vi "SP Convert Markers From Points.vi"(10 "Sweep":T8, 11 "Plot Control In":T1={"Trace Orientation"=enum."Overlay", "Frequency"={"Change Frequency"=FALSE, "Start"=500.0, "Stop"=1500.0, "Units"=enum."MHz"}, "Markers"=[], "Traces"=[]} {"Traces"."Reference" format="%#.2g"; "Traces"."Display Data" items=["Data", "Memory", "Data/Memory"]; "Traces"."Format" items=["Log Mag", "Phase", "Expanded Phase", "Delay", "Smith", "Polar", "Lin Mag", "SWR", "Loss", "Real", "Imaginary"]; "Traces"."Scale" min=0.001 step=1.0 format="%#.2g"; "Traces"."Position" min=0.0 max=10.0; "Frequency"."Stop" format="%.3g"; "Frequency"."Start" format="%.3g"}) -> (3 "Plot Control Out":T1={"Trace Orientation"=enum."Overlay", "Frequency"={"Change Frequency"=FALSE, "Start"=500.0, "Stop"=1500.0, "Units"=enum."MHz"}, "Markers"=[], "Traces"=[]} {"Traces"."Reference" format="%#.2g"; "Traces"."Display Data" items=["Data", "Memory", "Data/Memory"]; "Traces"."Format" items=["Log Mag", "Phase", "Expanded Phase", "Delay", "Smith", "Polar", "Lin Mag", "SWR", "Loss", "Real", "Imaginary"]; "Traces"."Scale" min=0.001 step=1.0 format="%#.2g"; "Traces"."Position" min=0.0 max=10.0; "Frequency"."Stop" format="%.3g"; "Frequency"."Start" format="%.3g"})   [LabVIEW 2011]
uses:
  TypeDefs/SP Frequency Units.ctl
  TypeDefs/SP Display Plot Controls Cluster.ctl
  TypeDefs/SP Marker Cluster.ctl
  TypeDefs/SP Marker Type.ctl
  TypeDefs/SP Display Trace Controls.ctl
  TypeDefs/SP Display Format.ctl
  TypeDefs/SP Display Data.ctl
panel:
  # "Div"
  # "Div"
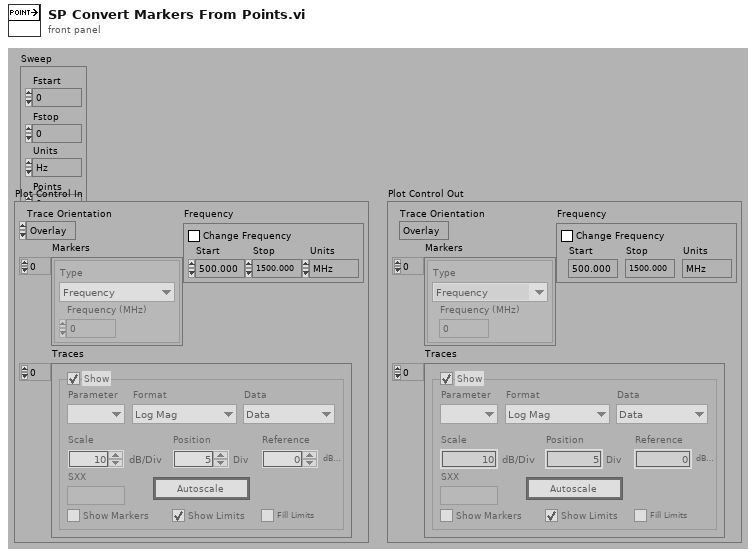
[diagram p1: front panel]
types:
  T1 = typedef "SP Display Plot Controls Cluster.ctl" = cluster{"Trace Orientation":enum32{"Overlay", "Split"}, "Frequency":cluster{"Change Frequency":bool, "Start":dbl, "Stop":dbl, "Units":T2}, "Markers":T3[], "Traces":T5[]}
  T2 = typedef "SP Frequency Units.ctl" = enum16{"Hz", "kHz", "MHz", "GHz", "Points"}
  T3 = typedef "SP Marker Cluster.ctl" = cluster{"Type":T4, "Frequency (MHz)":dbl}
  T4 = typedef "SP Marker Type.ctl" = enum16{"Frequency", "Trace Maximum", "Trace Minimum", "Limit Maximum", "Limit Minimum"}
  T5 = typedef "SP Display Trace Controls.ctl" = cluster{"Trace On":bool, "Measure":i32, "Format":T6, "Autoscale":bool, "Reference":dbl, "\nRefUnit":string, "Position":dbl, "Scale":dbl, "ScaleUnit":string, "LimitOn":bool, "LimitFill":bool, "Display Data":T7, "Show Markers":bool, "SXX":string}
  T6 = typedef "SP Display Format.ctl" = i32
  T7 = typedef "SP Display Data.ctl" = u16
  T8 = cluster{"Fstart":dbl, "Fstop":dbl, "Units":T2, "Points":i32}
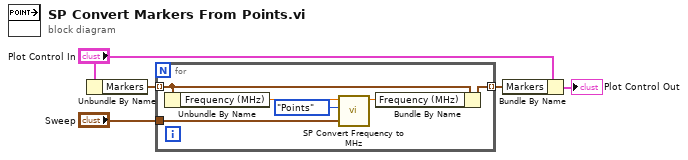
[diagram p0: block diagram]
diagram:
  n1 = Unbundle By Name("Plot Control In") -> ("Markers"=w2:T3[])
  n2 = for {
    tunnel: [w8] -> w3 mode=indexing
    tunnel: w2 -> [w9] mode=indexing
    tunnel: "Sweep" -> [w11]
    n3 = Unbundle By Name(w9) -> ("Frequency (MHz)"=w7:dbl)
    n4 = call "SP Convert Frequency to MHz.vi"("Sweep"=w11, "Units"=SP_Frequency_Units."Points", "Frequency"=w7) -> ("Converted Frequency"=w6:dbl)  [unwired: 8 out]
    n5 = Bundle By Name(cluster=w9, "Frequency (MHz)"=w6) -> (w8:T3)
  }
  n6 = Bundle By Name(cluster="Plot Control In", "Markers"=w3) -> (→"Plot Control Out":T1)
